vi "Get CD source file path.vi"(3 "CD Wizard - Internal Data":T1) -> (1 "CD Source file path":path)   [LabVIEW 2015]
doc: "Get the file path for the source folder. The source folder contains all created content like VIs, TypDefs, ..."
uses:
  TypDef/CD Wizard - Internal data.ctl
  TypDef/CD Wizard - Execution Mode.ctl
  TypDef/CD Wizard - Extra Page Name and GUID.ctl
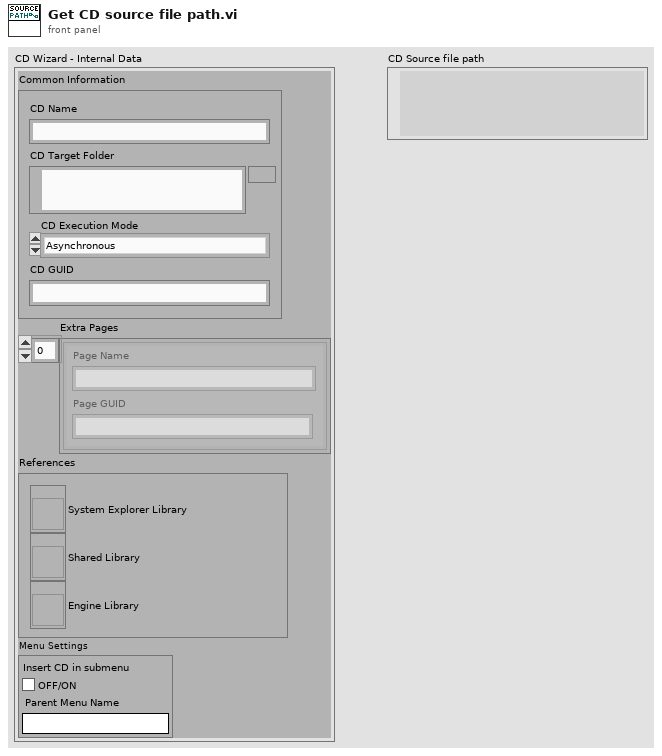
[diagram p1: front panel]
types:
  T1 = typedef "CD Wizard - Internal data.ctl" = cluster{"Common Information":cluster{"CD Name":string, "CD Target Folder":path, "CD Execution Mode":T2, "CD GUID":string}, "Extra Pages":T3[], "References":cluster{"System Explorer Library":refnum<vi>, "Shared Library":refnum<vi>, "Engine Library":refnum<vi>}, "Menu Settings":cluster{"Insert CD in submenu":bool, "Parent Menu Name":string}}
  T2 = typedef "CD Wizard - Execution Mode.ctl" = enum16{"Asynchronous", "Inline HW Interface", "Inline Model Interface", "Inline Timing and Sync", "Asynchronous Timing and Sync"}
  T3 = typedef "CD Wizard - Extra Page Name and GUID.ctl" = cluster{"Page Name":string, "Page GUID":string}
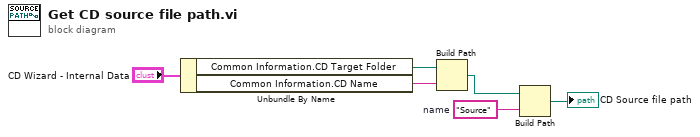
[diagram p0: block diagram]
diagram:
  w1 = "Source"  # name
  n1 = Unbundle By Name("CD Wizard - Internal Data") -> ("Common Information.CD Target Folder"=w5:path, "Common Information.CD Name"=w3:string)
  n2 = Build Path(base path=w5, name or relative path=w3) -> (appended path=w2:path)
  n3 = Build Path(base path=w2, name or relative path=w1) -> (appended path=→"CD Source file path":path)
